vi "2700电流加载及换向回读-PLC.vi"(0 "6510 in":refnum<visa-resource-name>, 1 "TDK in":refnum<visa-resource-name>, 2 "输入电流":dbl, 3 "Delay Time (s)":dbl=1.0 caption="延迟时间(s)", 4 "电源台数":u8=1, 5 "error in":errorcluster, 7 "y":dbl=5000.0 format="%#_13g") -> (6 "IsSuccess":bool, 14 "2700 out":refnum<visa-resource-name>, 15 "TDK out":refnum<visa-resource-name>, 16 "实际电流":dbl, 19 "error out":errorcluster)   [LabVIEW 2021]
uses:
  <instrlib>/Keithley 27XX/Public/Data/Read Single Point.vi
  <instrlib>/TDK-Lambda G Series/TDK-Lambda G Series.lvlib
  <instrlib>/Keithley 27XX/Keithley 27XX.lvlib
panel:
  out "x*y":dbl
  # "TDK 电流加载及换向"
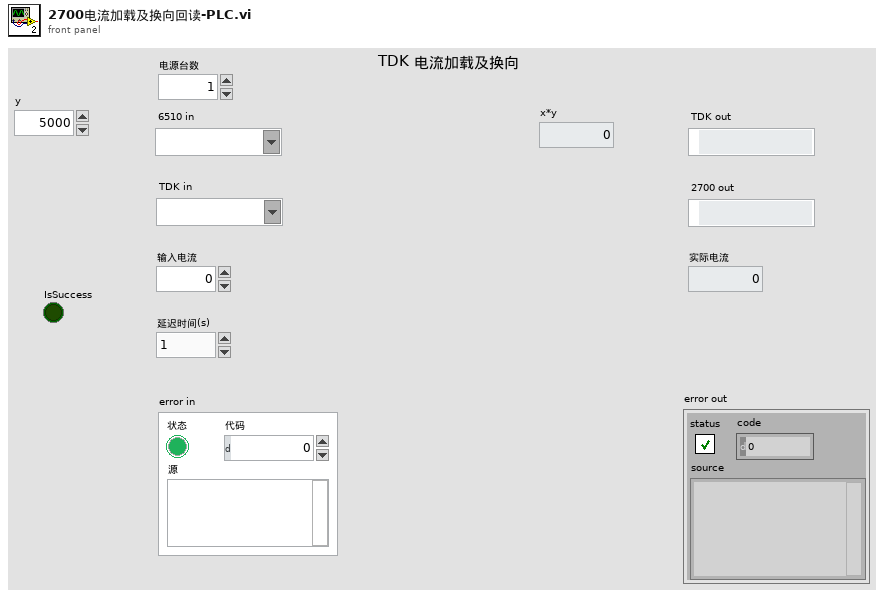
[diagram p1: front panel]
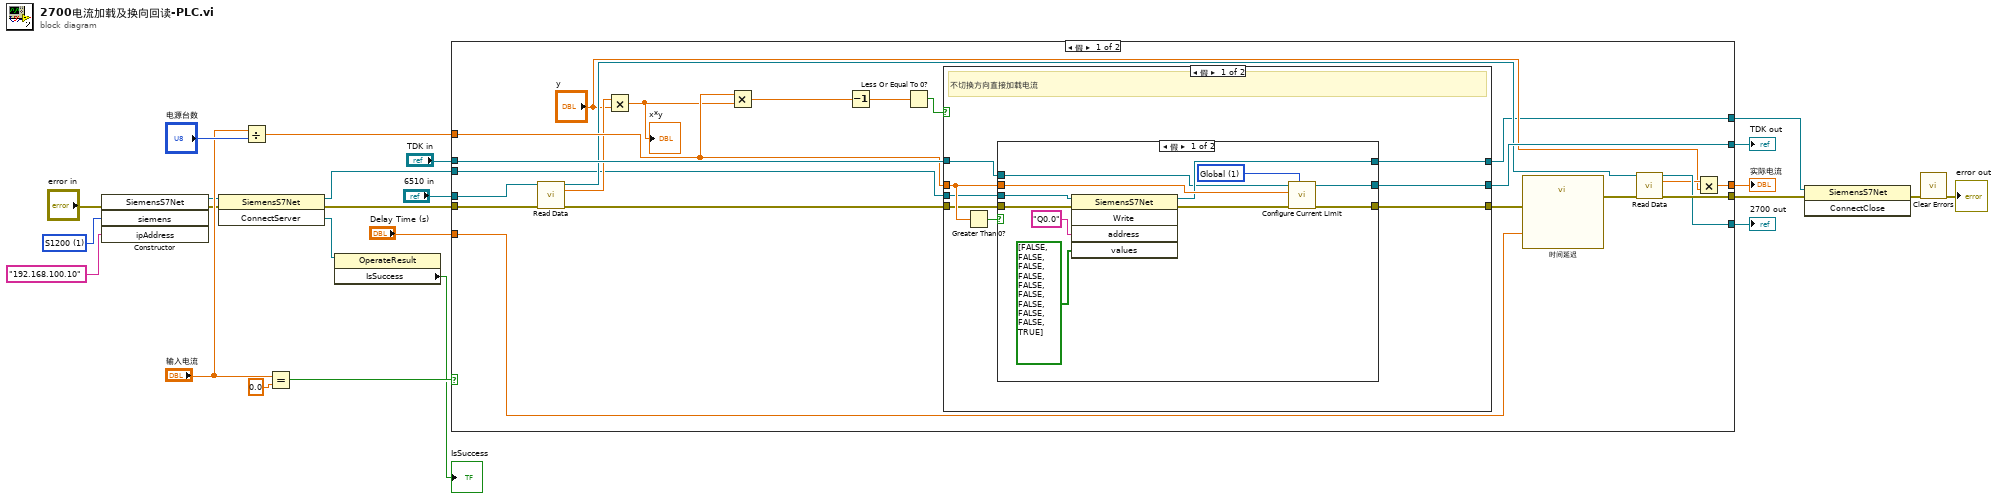
[diagram p0: block diagram]
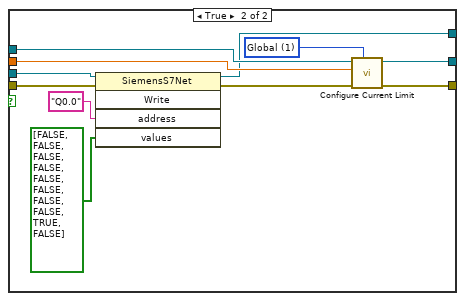
[diagram p2: hidden frame]
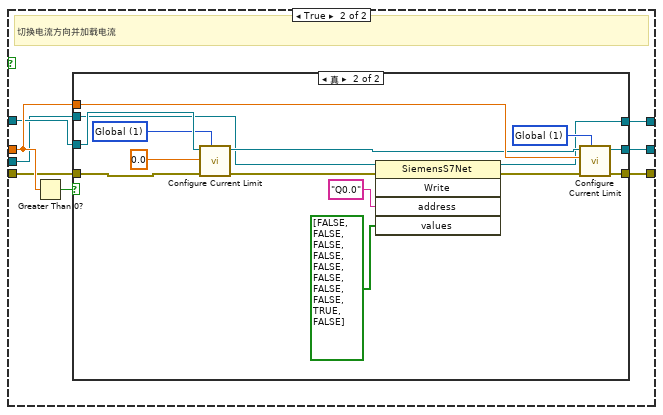
[diagram p3: hidden frame]
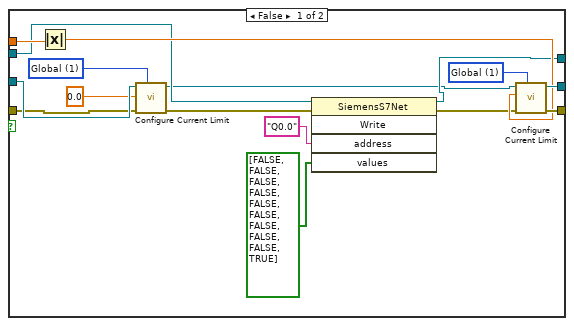
[diagram p4: hidden frame]
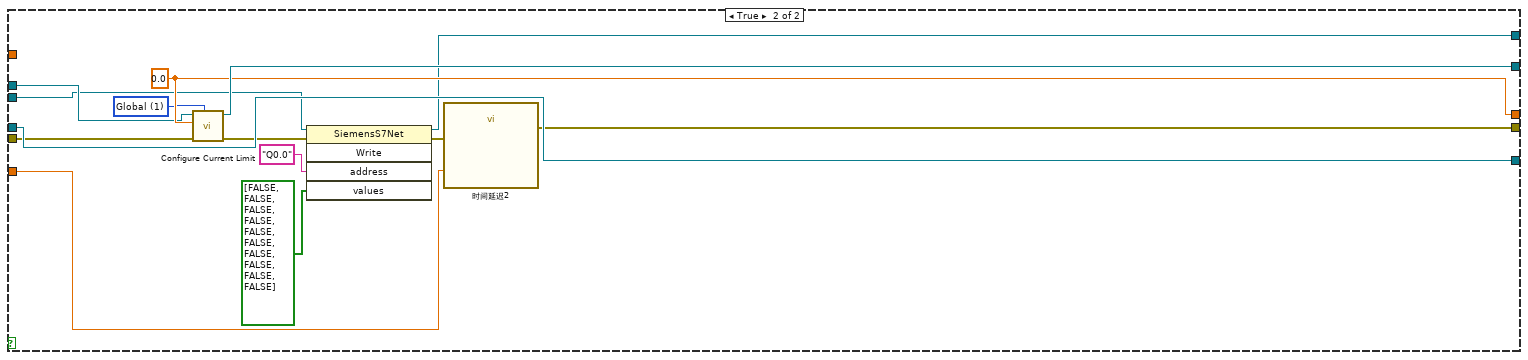
[diagram p5: hidden frame]
diagram:
  w12 = 1 items=["S1200"=1, "S300"=2, "S400"=3, "S1500"=4, "S200Smart"=5, "S200"=6] ("siemens")
  n1 = constructor class="SiemensS7Net"(error in="error in", "siemens"=w12, "ipAddress"="192.168.100.10") -> (reference out=w9:refnum<k24>, error out=w10:errorcluster)  [unwired: 2 in, 3 out]
  n2 = invoke class="SiemensS7Net" method="ConnectServer"(reference=w9, error in=w10) -> (reference out=w6:refnum<k24>, error out=w3:errorcluster, "ConnectServer"=w8:refnum<k24>)  [unwired: 1 in]
  n3 = Divide(x="输入电流", y="电源台数") -> (x/y=w14:dbl)
  n4 = Equal?(x="输入电流", y=0.0) -> (x = y?=w20:bool)
  n5 = property class="OperateResult"(reference=w8) -> ("IsSuccess"=→"IsSuccess":bool)  [unwired: 1 in, 2 out]
  n6 = case shown="假" w20 {
    tunnel: "TDK in" -> [w43 w125]
    tunnel: [w30 w123] -> w2
    tunnel: "Delay Time (s)" -> [w41 w122]
    tunnel: w3 -> [w34 w127]
    tunnel: [w40 w128] -> w22
    tunnel: "6510 in" -> [w35 w129]
    tunnel: [w29 w129] -> w18
    tunnel: w14 -> [w39 _]
    tunnel: [w37 w126] -> w19
    tunnel: w6 -> [w26 w119]
    tunnel: [w25 w118] -> w5
    frame False {
      n7 = call-poly <instrlib>:"Read Data.vi"("VISA resource name"=w35, "error in (no error)"=w34) -> ("VISA resource name out"=w32:refnum<visa-resource-name>, "Measurement Data"=w36:dbl, "error out"=w33:errorcluster)  [unwired: 11 in]
      n8 = Multiply(x=w36, y="y") -> (x*y=w38:dbl)
      "x*y" <- w38
      n9 = Multiply(x=w39, y=w38) -> (x*y=w45:dbl)
      n10 = Decrement(x=w45) -> (x-1=w44:dbl)
      n11 = Less Or Equal To 0?(x=w44) -> (x <= 0?=w46:bool)
      n12 = case shown="假" w46 {
        tunnel: w39 -> [w53 w84]
        tunnel: w33 -> [w50 w80]
        tunnel: w43 -> [w52 w82]
        tunnel: [w51 w81] -> w42
        tunnel: [w49 w79] -> w40
        tunnel: w26 -> [w47 w78]
        tunnel: [w48 w77] -> w25
        frame False {
          # "不切换方向直接加载电流"
          n13 = Greater Than 0?(x=w53) -> (x > 0?=w54:bool)
          n14 = case shown="假" w54 {
            tunnel: w53 -> [w61 w74]
            tunnel: w52 -> [w56 w75]
            tunnel: [w64 w73] -> w51
            tunnel: w50 -> [w55 w71]
            tunnel: [w65 w76] -> w49
            tunnel: [w60 w69] -> w48
            tunnel: w47 -> [w57 w66]
            frame False {
              w63 = u16 1 items=["Single", "Global"] ("Globalize (0: Single)")
              n15 = invoke class="SiemensS7Net" method="Write"(reference=w57, error in=w55, "address"="Q0.0", "values"=bool[] [FALSE, FALSE, FALSE, FALSE, FALSE, FALSE, FALSE, FALSE, FALSE, TRUE]) -> (reference out=w60:refnum<k24>, error out=w62:errorcluster)  [unwired: 1 in, 3 out]
              n16 = call <instrlib>:"Configure Current Limit.vi"("Globalize (0: Single)"=w63, "error in (no error)"=w62, "Current Limit (0A)"=w61, "VISA resource name"=w56) -> ("error out"=w64:errorcluster, "VISA resource name out"=w65:refnum<visa-resource-name>)  [unwired: 6 in]
            }
            frame True {
              w72 = u16 1 items=["Single", "Global"] ("Globalize (0: Single)")
              n17 = invoke class="SiemensS7Net" method="Write"(reference=w66, error in=w71, "address"="Q0.0", "values"=bool[] [FALSE, FALSE, FALSE, FALSE, FALSE, FALSE, FALSE, FALSE, TRUE, FALSE]) -> (reference out=w69:refnum<k24>, error out=w70:errorcluster)  [unwired: 1 in, 3 out]
              n18 = call <instrlib>:"Configure Current Limit.vi"("Globalize (0: Single)"=w72, "error in (no error)"=w70, "Current Limit (0A)"=w74, "VISA resource name"=w75) -> ("error out"=w73:errorcluster, "VISA resource name out"=w76:refnum<visa-resource-name>)  [unwired: 6 in]
            }
          }
        }
        frame True {
          # "切换电流方向并加载电流"
          n19 = Greater Than 0?(x=w84) -> (x > 0?=w83:bool)
          n20 = case shown="真" w83 {
            tunnel: w84 -> [w100 w113]
            tunnel: w82 -> [w96 w112]
            tunnel: [w99 w115] -> w81
            tunnel: w80 -> [w94 w110]
            tunnel: [w98 w114] -> w79
            tunnel: w78 -> [w91 w101]
            tunnel: [w90 w102] -> w77
            frame False {
              w92 = u16 1 items=["Single", "Global"] ("Globalize (0: Single)")
              w93 = u16 1 items=["Single", "Global"] ("Globalize (0: Single)")
              n21 = Absolute Value(x=w100) -> (abs(x)=w97:dbl)
              n22 = call <instrlib>:"Configure Current Limit.vi"("Globalize (0: Single)"=w92, "error in (no error)"=w94, "Current Limit (0A)"=0.0 ("Curr(0)"), "VISA resource name"=w96) -> ("error out"=w89:errorcluster, "VISA resource name out"=w85:refnum<visa-resource-name>)  [unwired: 6 in]
              n23 = invoke class="SiemensS7Net" method="Write"(reference=w91, error in=w89, "address"="Q0.0", "values"=bool[] [FALSE, FALSE, FALSE, FALSE, FALSE, FALSE, FALSE, FALSE, FALSE, TRUE]) -> (reference out=w90:refnum<k24>, error out=w88:errorcluster)  [unwired: 1 in, 3 out]
              n24 = call <instrlib>:"Configure Current Limit.vi"("Globalize (0: Single)"=w93, "error in (no error)"=w88, "Current Limit (0A)"=w97, "VISA resource name"=w85) -> ("error out"=w99:errorcluster, "VISA resource name out"=w98:refnum<visa-resource-name>)  [unwired: 6 in]
            }
            frame True {
              w107 = u16 1 items=["Single", "Global"] ("Globalize (0: Single)")
              w108 = u16 1 items=["Single", "Global"] ("Globalize (0: Single)")
              n25 = call <instrlib>:"Configure Current Limit.vi"("Globalize (0: Single)"=w107, "error in (no error)"=w110, "Current Limit (0A)"=0.0 ("Curr(0)"), "VISA resource name"=w112) -> ("error out"=w106:errorcluster, "VISA resource name out"=w109:refnum<visa-resource-name>)  [unwired: 6 in]
              n26 = invoke class="SiemensS7Net" method="Write"(reference=w101, error in=w106, "address"="Q0.0", "values"=bool[] [FALSE, FALSE, FALSE, FALSE, FALSE, FALSE, FALSE, FALSE, TRUE, FALSE]) -> (reference out=w102:refnum<k24>, error out=w105:errorcluster)  [unwired: 1 in, 3 out]
              n27 = call <instrlib>:"Configure Current Limit.vi"("Globalize (0: Single)"=w108, "error in (no error)"=w105, "Current Limit (0A)"=w113, "VISA resource name"=w109) -> ("error out"=w115:errorcluster, "VISA resource name out"=w114:refnum<visa-resource-name>)  [unwired: 6 in]
            }
          }
        }
      }
      n28 = call "时间延迟"("error in (no error)"=w42, "Delay Time (s)"=w41) -> ("error out"=w31:errorcluster)  [unwired: 9 in]
      n29 = call-poly <instrlib>:"Read Data.vi"("VISA resource name"=w32, "error in (no error)"=w31) -> ("VISA resource name out"=w29:refnum<visa-resource-name>, "Measurement Data"=w28:dbl, "error out"=w30:errorcluster)  [unwired: 11 in]
      n30 = Multiply(x=w28, y="y") -> (x*y=w37:dbl)
    }
    frame True {
      w124 = u16 1 items=["Single", "Global"] ("Globalize (0: Single)")
      w126 = 0.0 ("Curr(0)")
      n31 = call <instrlib>:"Configure Current Limit.vi"("Globalize (0: Single)"=w124, "error in (no error)"=w127, "Current Limit (0A)"=w126, "VISA resource name"=w125) -> ("error out"=w120:errorcluster, "VISA resource name out"=w128:refnum<visa-resource-name>)  [unwired: 6 in]
      n32 = invoke class="SiemensS7Net" method="Write"(reference=w119, error in=w120, "address"="Q0.0", "values"=bool[] [FALSE, FALSE, FALSE, FALSE, FALSE, FALSE, FALSE, FALSE, FALSE, FALSE]) -> (reference out=w118:refnum<k24>, error out=w121:errorcluster)  [unwired: 1 in, 3 out]
      n33 = call "时间延迟2"("error in (no error)"=w121, "Delay Time (s)"=w122) -> ("error out"=w123:errorcluster)  [unwired: 9 in]
    }
  }
  "实际电流" <- w19
  "TDK out" <- w22
  "2700 out" <- w18
  n34 = invoke class="SiemensS7Net" method="ConnectClose"(reference=w5, error in=w2) -> (error out=w1:errorcluster)  [unwired: 1 in, 2 out]
  n35 = call <vilib>:"Clear Errors.vi"("error in (no error)"=w1) -> ("error out"=→"error out":errorcluster)  [unwired: 5 in, 1 out]
